vi "Cannon Limit Switch Update.vi"(1 "Cannon Info In":T2) -> (0 "Cannon Info Out?":T2)   [LabVIEW 2013]
uses:
  <vilib>/Rock Robotics/WPI/Solenoid/WPI_SolenoidValue.ctl
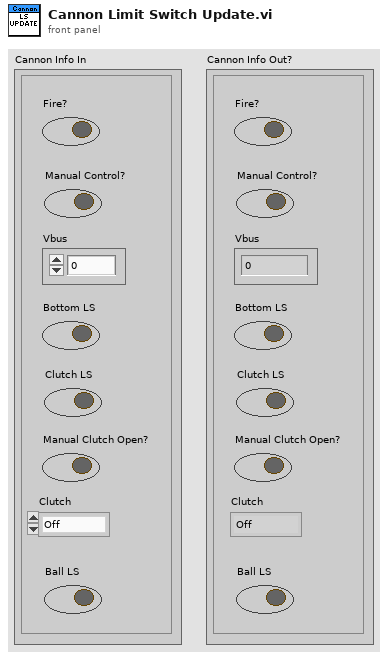
[diagram p1: front panel]
types:
  T1 = typedef "WPI_SolenoidValue.ctl" = enum16{"Off", "On", "Forward", "Reverse"}
  T2 = cluster{"Fire?":bool, "Manual Control?":bool, "Vbus":dbl, "Bottom LS":bool, "Clutch LS ":bool, "Manual Clutch Open?":bool, "Clutch":T1, "Ball LS":bool}
  T3 = typedef "WPI_DigitalInputDevRef.ctl" = cluster{"DevStatus":errorcluster, "DIO Channel":T4, "Digital Module":T5}
  T4 = typedef "FPGA_DIOChannel.ctl" = enum8{"DIO 1", "DIO 2", "DIO 3", "DIO 4", "DIO 5", "DIO 6", "DIO 7", "DIO 8", "DIO 9", "DIO 10", "DIO 11", "DIO 12", "DIO 13", "DIO 14", "Invalid"}
  T5 = typedef "FPGA_TypedefDigitalModule.ctl" = enum16{"Digital Module 1", "Digital Module 2"}
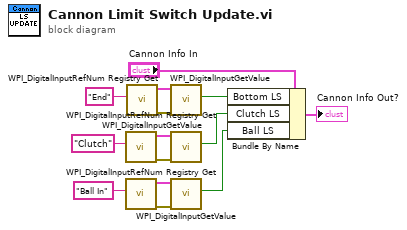
[diagram p0: block diagram]
diagram:
  n1 = call <vilib>:"WPI_DigitalInputRefNum Registry Get.vi"("refnum name"="Clutch") -> ("error out"=w11:errorcluster, "DigitalInputDevRef"=w10:T3)  [unwired: 9 in]
  n2 = call <vilib>:"WPI_DigitalInputRefNum Registry Get.vi"("refnum name"="Ball In") -> ("error out"=w7:errorcluster, "DigitalInputDevRef"=w6:T3)  [unwired: 9 in]
  n3 = call <vilib>:"WPI_DigitalInputRefNum Registry Get.vi"("refnum name"="End") -> ("error out"=w9:errorcluster, "DigitalInputDevRef"=w8:T3)  [unwired: 9 in]
  n4 = call <vilib>:"WPI_DigitalInputGetValue.vi"("error in (no error)"=w9, "DigitalInputDevRef"=w8) -> ("Value"=w3:bool)  [unwired: 7 in, 2 out]
  n5 = call <vilib>:"WPI_DigitalInputGetValue.vi"("error in (no error)"=w11, "DigitalInputDevRef"=w10) -> ("Value"=w1:bool)  [unwired: 7 in, 2 out]
  n6 = call <vilib>:"WPI_DigitalInputGetValue.vi"("error in (no error)"=w7, "DigitalInputDevRef"=w6) -> ("Value"=w2:bool)  [unwired: 7 in, 2 out]
  n7 = Bundle By Name(cluster="Cannon Info In", "Bottom LS"=w3, "Clutch LS"=w1, "Ball LS"=w2) -> (→"Cannon Info Out?":T2)
